vi "Live Pulse Counter.vi"(10 "Trajanje merenja pulsa (s)":i32, 11 "Filtered X":dbl[](array[numeric])) -> (3 "Numeric":dbl)   [LabVIEW 2018]
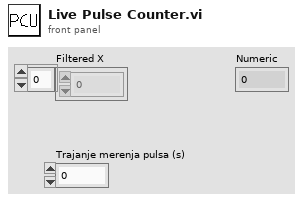
[diagram p1: front panel]
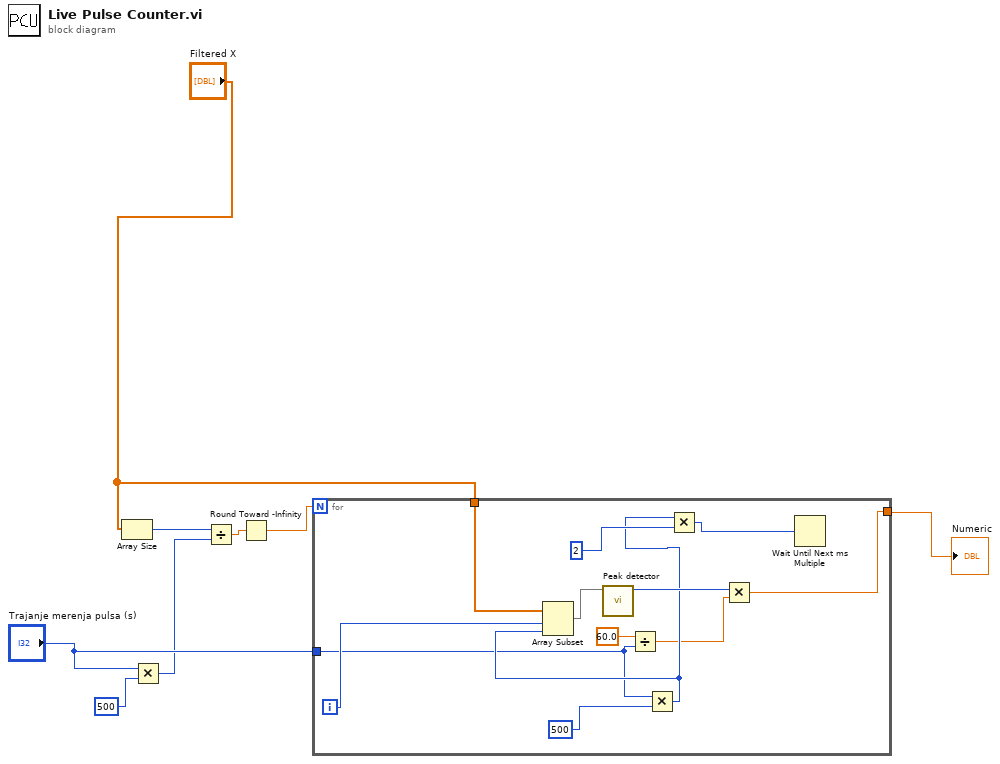
[diagram p0: block diagram]
diagram:
  n1 = Array Size(array="Filtered X") -> (size(s)=w1:i32)
  n2 = Multiply(x="Trajanje merenja pulsa (s)", y=500) -> (x*y=w5:i32)
  n3 = Divide(x=w1, y=w5) -> (x/y=w2:dbl)
  n4 = Round Toward -Infinity(1:w2) -> (0:w3:dbl)
  n5 = for {
    N: w3 -> [_]
    tunnel: [w11] -> w6
    tunnel: "Trajanje merenja pulsa (s)" -> [w10]
    tunnel: "Filtered X" -> [w9]
    i -> [w20]
    n6 = Divide(x=60.0, y=w10) -> (x/y=w12:dbl)
    n7 = Multiply(x=w10, y=500) -> (x*y=w15:i32)
    n8 = Array Subset(array=w9, index=w20, length=w15) -> (w19:dbl[])
    n9 = call "Peak detector.vi"("Filtered X"=w19) -> ("Numeric"=w18:i32)  [unwired: 10 in]
    n10 = Multiply(x=w15, y=2) -> (x*y=w14:i32)
    n11 = Multiply(x=w18, y=w12) -> (x*y=w11:dbl)
    n12 = Wait Until Next ms Multiple(millisecond multiple=w14) -> ()  [unwired: 1 out]
  }
  "Numeric" <- w6
